vi "LV_ATS.vi"(5 "test json in":string) -> (0 "formatted test json out":string, 1 "ats json out":string, 2 "PASS":bool, 3 "error out":errorcluster)   [LabVIEW 2019]
panel:
  out "error out 2":errorcluster
  in  "ats json in":string
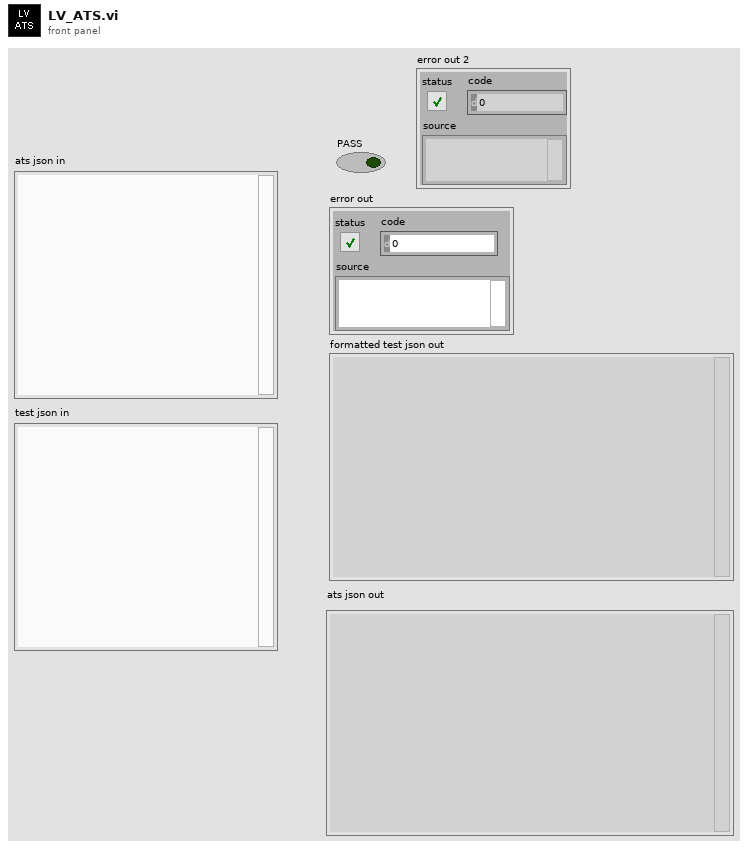
[diagram p1: front panel]
types:
  T1 = enum16{"open", "replace", "create", "open or create", "replace or create", "replace or create with confirmation"}
  T2 = cluster{"description":string, "error type":enum32{"generic failure", "boundary case", "precision", "expected error"}}[]
  T3 = cluster{"control\nname":string, "type\ndescriptor":i16[], "flattened\ndata":string}[]
  T4 = cluster{"Load time (ms)":u32, "DataSize after execution":u32, "Execute time":u32, "DataSize before execution":u32}
  T5 = cluster{"array of error description":cluster{"description":string, "error type":string}[], "outputs":cluster{"control\nname":string, "type\ndescriptor":i16[], "flattened\ndata":string}[], "error out 2":errorcluster, "Metrics":cluster{"Load time (ms)":u32, "DataSize after execution":u32, "Execute time":u32, "DataSize before execution":u32}, "array output?":bool}
  T6 = cluster{"description":string, "error type":string}[]
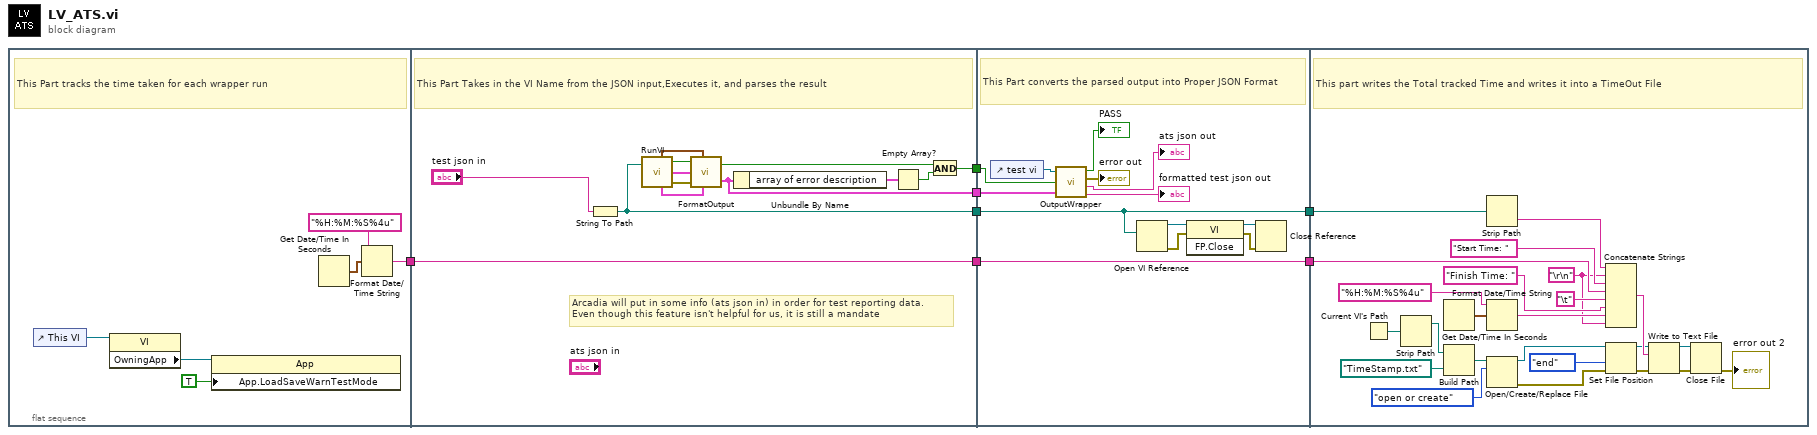
[diagram p0: block diagram]
diagram:
  n1 = flat-sequence {
    tunnel: [w11] -> w5
    tunnel: [w24] -> w7
    tunnel: [w26] -> w6
    tunnel: w5 -> [w21]
    tunnel: [w21] -> w4
    tunnel: [w20] -> w2
    tunnel: w7 -> [w37]
    tunnel: w6 -> [w38]
    tunnel: w4 -> [w32]
    tunnel: [w32] -> w3
    tunnel: w2 -> [w31]
    tunnel: [w31] -> w1
    tunnel: w3 -> [w44]
    tunnel: w1 -> [w54]
    frame #0 {
      # "This Part tracks the time taken for each wrapper run"
      n2 = control-ref of="This VI"() -> (w10:refnum<vi>)
      n3 = property class="VI"(reference=w10) -> ("OwningApp"=w9:refnum<vi>)  [unwired: 1 in, 2 out]
      n4 = property class="App"(reference=w9, "App.LoadSaveWarnTestMode"=TRUE ("Load and Save Warnings:Auto Test Mode")) -> ()  [unwired: 1 in, 2 out]
      n5 = Get Date/Time In Seconds() -> (seconds since 1Jan1904=w13:timestamp)
      n6 = Format Date/Time String(time format string (%c)="%H:%M:%S%4u", seconds (now)=w13) -> (date/time string=w11:string)  [unwired: 1 in]
    }
    frame #1 {
      # "Arcadia will put in some info (ats json in) in order for test reporting data.\nEven though this feature isn't helpful for us, it is still a mandate"
      # "This Part Takes in the VI Name from the JSON input,Executes it, and parses the result"
      n7 = String To Path(string="test json in") -> (path=w20:path)
      n8 = call "RunVI.vi"("VI path"=w20) -> ("error out"=w16:errorcluster, "array of error description"=w15:T2, "outputs"=w17:T3, "array output?"=w18:bool, "Metrics"=w19:T4)  [unwired: 1 in]
      n9 = call "FormatOutput.vi"("array output?"=w18, "Metrics"=w19, "outputs"=w17, "error out 2"=w16, "array of error description"=w15) -> ("Pass"=w25:bool, "FinalCluster"=w24:T5)
      n10 = Unbundle By Name(w24) -> ("array of error description"=w23:T6)
      n11 = Empty Array?(array=w23) -> (empty?=w22:bool)
      n12 = And(x=w25, y=w22) -> (x .and. y?=w26:bool)
    }
    frame #2 {
      # "This Part converts the parsed output into Proper JSON Format"
      n13 = control-ref of="test vi"() -> (w39:refnum<vi>)
      n14 = call "OutputWrapper.vi"("VI in"=w39, "pass"=w38, "FinalCluster"=w37) -> ("PASS"=→"PASS":bool, "error out"=→"error out":errorcluster, "ats json out"=→"ats json out":string, "formatted test json out"=→"formatted test json out":string)
      n15 = Open VI Reference(vi path=w31) -> (vi reference=w30:refnum<vi>, error out=w29:errorcluster)  [unwired: 5 in]
      n16 = invoke class="VI" method="FP.Close"(reference=w30, error in=w29) -> (reference out=w27:refnum<vi>, error out=w28:errorcluster)  [unwired: 1 in, 1 out]
      n17 = Close Reference(reference=w27, error in (no error)=w28) -> ()  [unwired: 1 out]
    }
    frame #3 {
      w40 = "\r\n"
      # "This part writes the Total tracked Time and writes it into a TimeOut File"
      n18 = Current VI's Path() -> (path=w52:path)
      n19 = Strip Path(path=w52) -> (stripped path=w51:path)  [unwired: 1 out]
      n20 = Get Date/Time In Seconds() -> (seconds since 1Jan1904=w62:timestamp)
      n21 = Build Path(base path=w51, name or relative path=path "TimeStamp.txt") -> (appended path=w55:path)
      n22 = Strip Path(path=w54) -> (name=w53:string)  [unwired: 1 out]
      n23 = Format Date/Time String(time format string (%c)="%H:%M:%S%4u", seconds (now)=w62) -> (date/time string=w41:string)  [unwired: 1 in]
      n24 = Open/Create/Replace File(file path (use dialog)=w55, operation (0:open)=T1."open or create") -> (refnum out=w50:refnum<file>, error out=w49:errorcluster)  [unwired: 4 in, 1 out]
      n25 = Concatenate Strings(w53, w40, "Start Time: " ("string"), w44, "\t", "Finish Time: " ("string"), w41, w40) -> (w60:string)
      n26 = Set File Position(refnum=w50, from (0:start)=enum16{"start", "end", "current"}."end", error in=w49) -> (refnum out=w47:refnum<file>, error out=w46:errorcluster)  [unwired: 1 in]
      n27 = Write to Text File(file (use dialog)=w47, text=w60, error in=w46) -> (refnum out=w59:refnum<file>, error out=w58:errorcluster)  [unwired: 1 in, 1 out]
      n28 = Close File(refnum=w59, error in=w58) -> (error out=→"error out 2":errorcluster)  [unwired: 1 out]
    }
  }
